vi "Read A.vi"(8 "error in (no error)":errorcluster, 11 "My Custom Type in":refnum<class "My Custom Type.lvclass">) -> (0 "error out":errorcluster, 2 "fieldA":i32, 3 "My Custom Type out":refnum<class "My Custom Type.lvclass">)   [LabVIEW 2020, in "My Custom Type.lvclass"]
uses:
  My Custom Type.lvclass
  My Custom Type.lvclass/My Custom Type.ctl
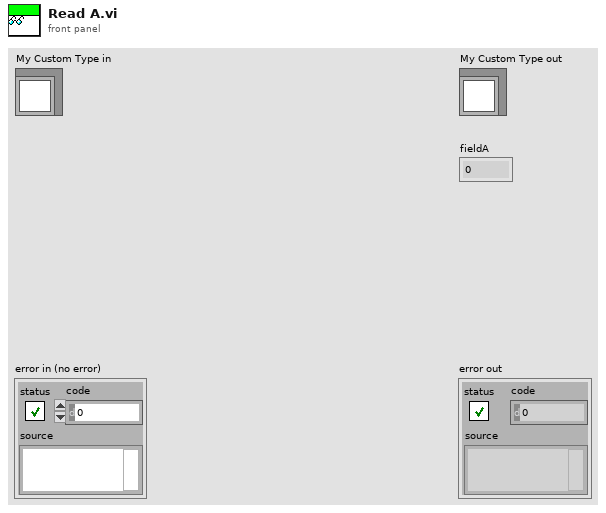
[diagram p1: front panel]
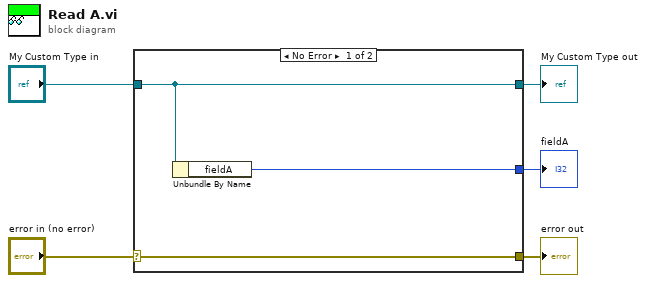
[diagram p0: block diagram]
diagram:
  n1 = case shown="No Error" "error in (no error)" {
    selector: "error in (no error)" -> [w8 w9]
    tunnel: [w8 w9] -> w4
    tunnel: [w6 w10] -> w2
    tunnel: "My Custom Type in" -> [w6 w10]
    tunnel: [w7 _] -> w1
    frame No Error {
      n2 = Unbundle By Name(w6) -> ("fieldA"=w7:i32)
    }
    frame Error {
    }
  }
  "error out" <- w4
  "My Custom Type out" <- w2
  "fieldA" <- w1
